vi "Deserialize Object (XML).vi"(8 "error in":errorcluster, 9 "key-value-type in":T1[](array[typedef]), 11 "object type":refnum<class "_ISerializable.lvclass">) -> (0 "casting error":errorcluster, 3 "object out":refnum<class "_ISerializable.lvclass">)   [LabVIEW 2018, in "Serializer.lvclass"]
uses:
  Serializer.lvclass
  _Serializable Base Object/_ISerializable.lvclass
  Typedefs/key-value-type cluster.ctl
  <vilib>/xml/Close Reference(Node).vi
  <resource>/objmgr/DOMUserDefRef.rc
  <vilib>/xml/NI_XML.lvlib
  <vilib>/Analysis/NI_AALBase.lvlib
  ORM Scripter/ORM Scripter.lvclass
  <vilib>/Analysis/baseanly.llb/Mean (DBL).vi
panel:
  out "error out":errorcluster
  out "XML-Pretty":string
  out "Generated XML":string
  out "default object xml string":string
  # "<Object>\n<Name>object in</Name>\n<NumLevels>2</NumLevels>\n<Class>DataTypes.lvclass</Class>\n<Version>1.0.0.4</Version>\n<Version>1.0.0.1</Version>\n<Cluster>\n</Cluster>\n<Cluster>\n<Name>DataTypes.lvclass</Name>\n<NumElts>17</NumElts>\n<Boolean>\n<Name>Boolean</Name>\n<Val>0</Val>\n</Boolean>\n<String>\n<Name>String</Name>\n<Val>STRING DATA</Val>\n</String>\n<U16>\n<Name>Ring</Name>\n<Val>1</Val>\n</U16>\n<EW>\n<Name>Enum</Name>\n<Choice>enum-value-0</Choice>\n<Choice>enum-value-1</Choice>\n<Choice>enum-value-2</Choice>\n<Val>2</Val>\n</EW>\n<DBL>\n<Name>Numeric DBL</Name>\n<Val>0.36114694623797</Val>\n</DBL>\n<SGL>\n<Name>Numeric SGL</Name>\n<Val>0.36115</Val>\n</SGL>\n<CDB>\n<Name>Numeric C-DBL</Name>\n<Val>0.36114694623797 +0.00000000000000 i</Val>\n</CDB>\n<CSG>\n<Name>Numeric C-SGL</Name>\n<Val>0.36115 +0.00000 i</Val>\n</CSG>\n<U8>\n<Name>Numeric U8</Name>\n<Val>33</Val>\n</U8>\n<I8>\n<Name>Numeric I8</Name>\n<Val>30</Val>\n</I8>\n<U16>\n<Name>Numeric U16</Name>\n<Val>28</Val>\n</U16>\n<I16>\n<Name>Numeric I16</Name>\n<Val>50</Val>\n</I16>\n<U32>\n<Name>Numeric U32</Name>\n<Val>68</Val>\n</U32>\n<I32>\n<Name>Numeric I32</Name>\n<Val>54</Val>\n</I32>\n<U64>\n<Name>Numeric U64</Name>\n<Val>45</Val>\n</U64>\n<I64>\n<Name>Numeric I64</Name>\n<Val>29</Val>\n</I64>\n<Timestamp>\n<Name>Time Stamp</Name>\n<Cluster>\n<Name></Name>\n<NumElts>4</NumElts>\n<I32>\n<Name></Name>\n<Val>0</Val>\n</I32>\n<I32>\n<Name></Name>\n<Val>632510464</Val>\n</I32>\n<I32>\n<Name></Name>\n<Val>-640183486</Val>\n</I32>\n<I32>\n<Name></Name>\n<Val>0</Val>\n</I32>\n</Cluster>\n</Timestamp>\n</Cluster>\n</Object>"
  # "<Object>\n<Name>object type</Name>\n<NumLevels>2</NumLevels>\n<Class>DataTypes.lvclass</Class>\n<Version>1.0.0.4</Version>\n<Version>1.0.0.1</Version>\n<Cluster>\n<Name>DataTypes.lvclass</Name>\n<NumElts>17</NumElts>\n<Boolean>\n<Name>Boolean</Name>\n<Val>0</Val>\n</Boolean>\n<String>\n<Name>String</Name>\n<Val>STRING DATA</Val>\n</String>\n<U16>\n<Name>Ring</Name>\n<Val>1</Val>\n</U16>\n<EW>\n<Name>Enum</Name>\n<Choice>enum-value-0</Choice>\n<Choice>enum-value-1</Choice>\n<Choice>enum-value-2</Choice>\n<Val>2</Val>\n</EW>\n<DBL>\n<Name>Numeric DBL</Name>\n<Val>0.69305757967832</Val>\n</DBL>\n<SGL>\n<Name>Numeric SGL</Name>\n<Val>0.69306</Val>\n</SGL>\n<CDB>\n<Name>Numeric C-DBL</Name>\n<Val>0.69305757967832 +0.00000000000000 i</Val>\n</CDB>\n<CSG>\n<Name>Numeric C-SGL</Name>\n<Val>0.69306 +0.00000 i</Val>\n</CSG>\n<U8>\n<Name>Numeric U8</Name>\n<Val>90</Val>\n</U8>\n<I8>\n<Name>Numeric I8</Name>\n<Val>84</Val>\n</I8>\n<U16>\n<Name>Numeric U16</Name>\n<Val>4</Val>\n</U16>\n<I16>\n<Name>Numeric I16</Name>\n<Val>41</Val>\n</I16>\n<U32>\n<Name>Numeric U32</Name>\n<Val>91</Val>\n</U32>\n<I32>\n<Name>Numeric I32</Name>\n<Val>70</Val>\n</I32>\n<U64>\n<Name>Numeric U64</Name>\n<Val>48</Val>\n</U64>\n<I64>\n<Name>Numeric I64</Name>\n<Val>30</Val>\n</I64>\n<Timestamp>\n<Name>Time Stamp</Name>\n<Val>\n</Val>\n</Timestamp>\n</Cluster>\n</Object>"
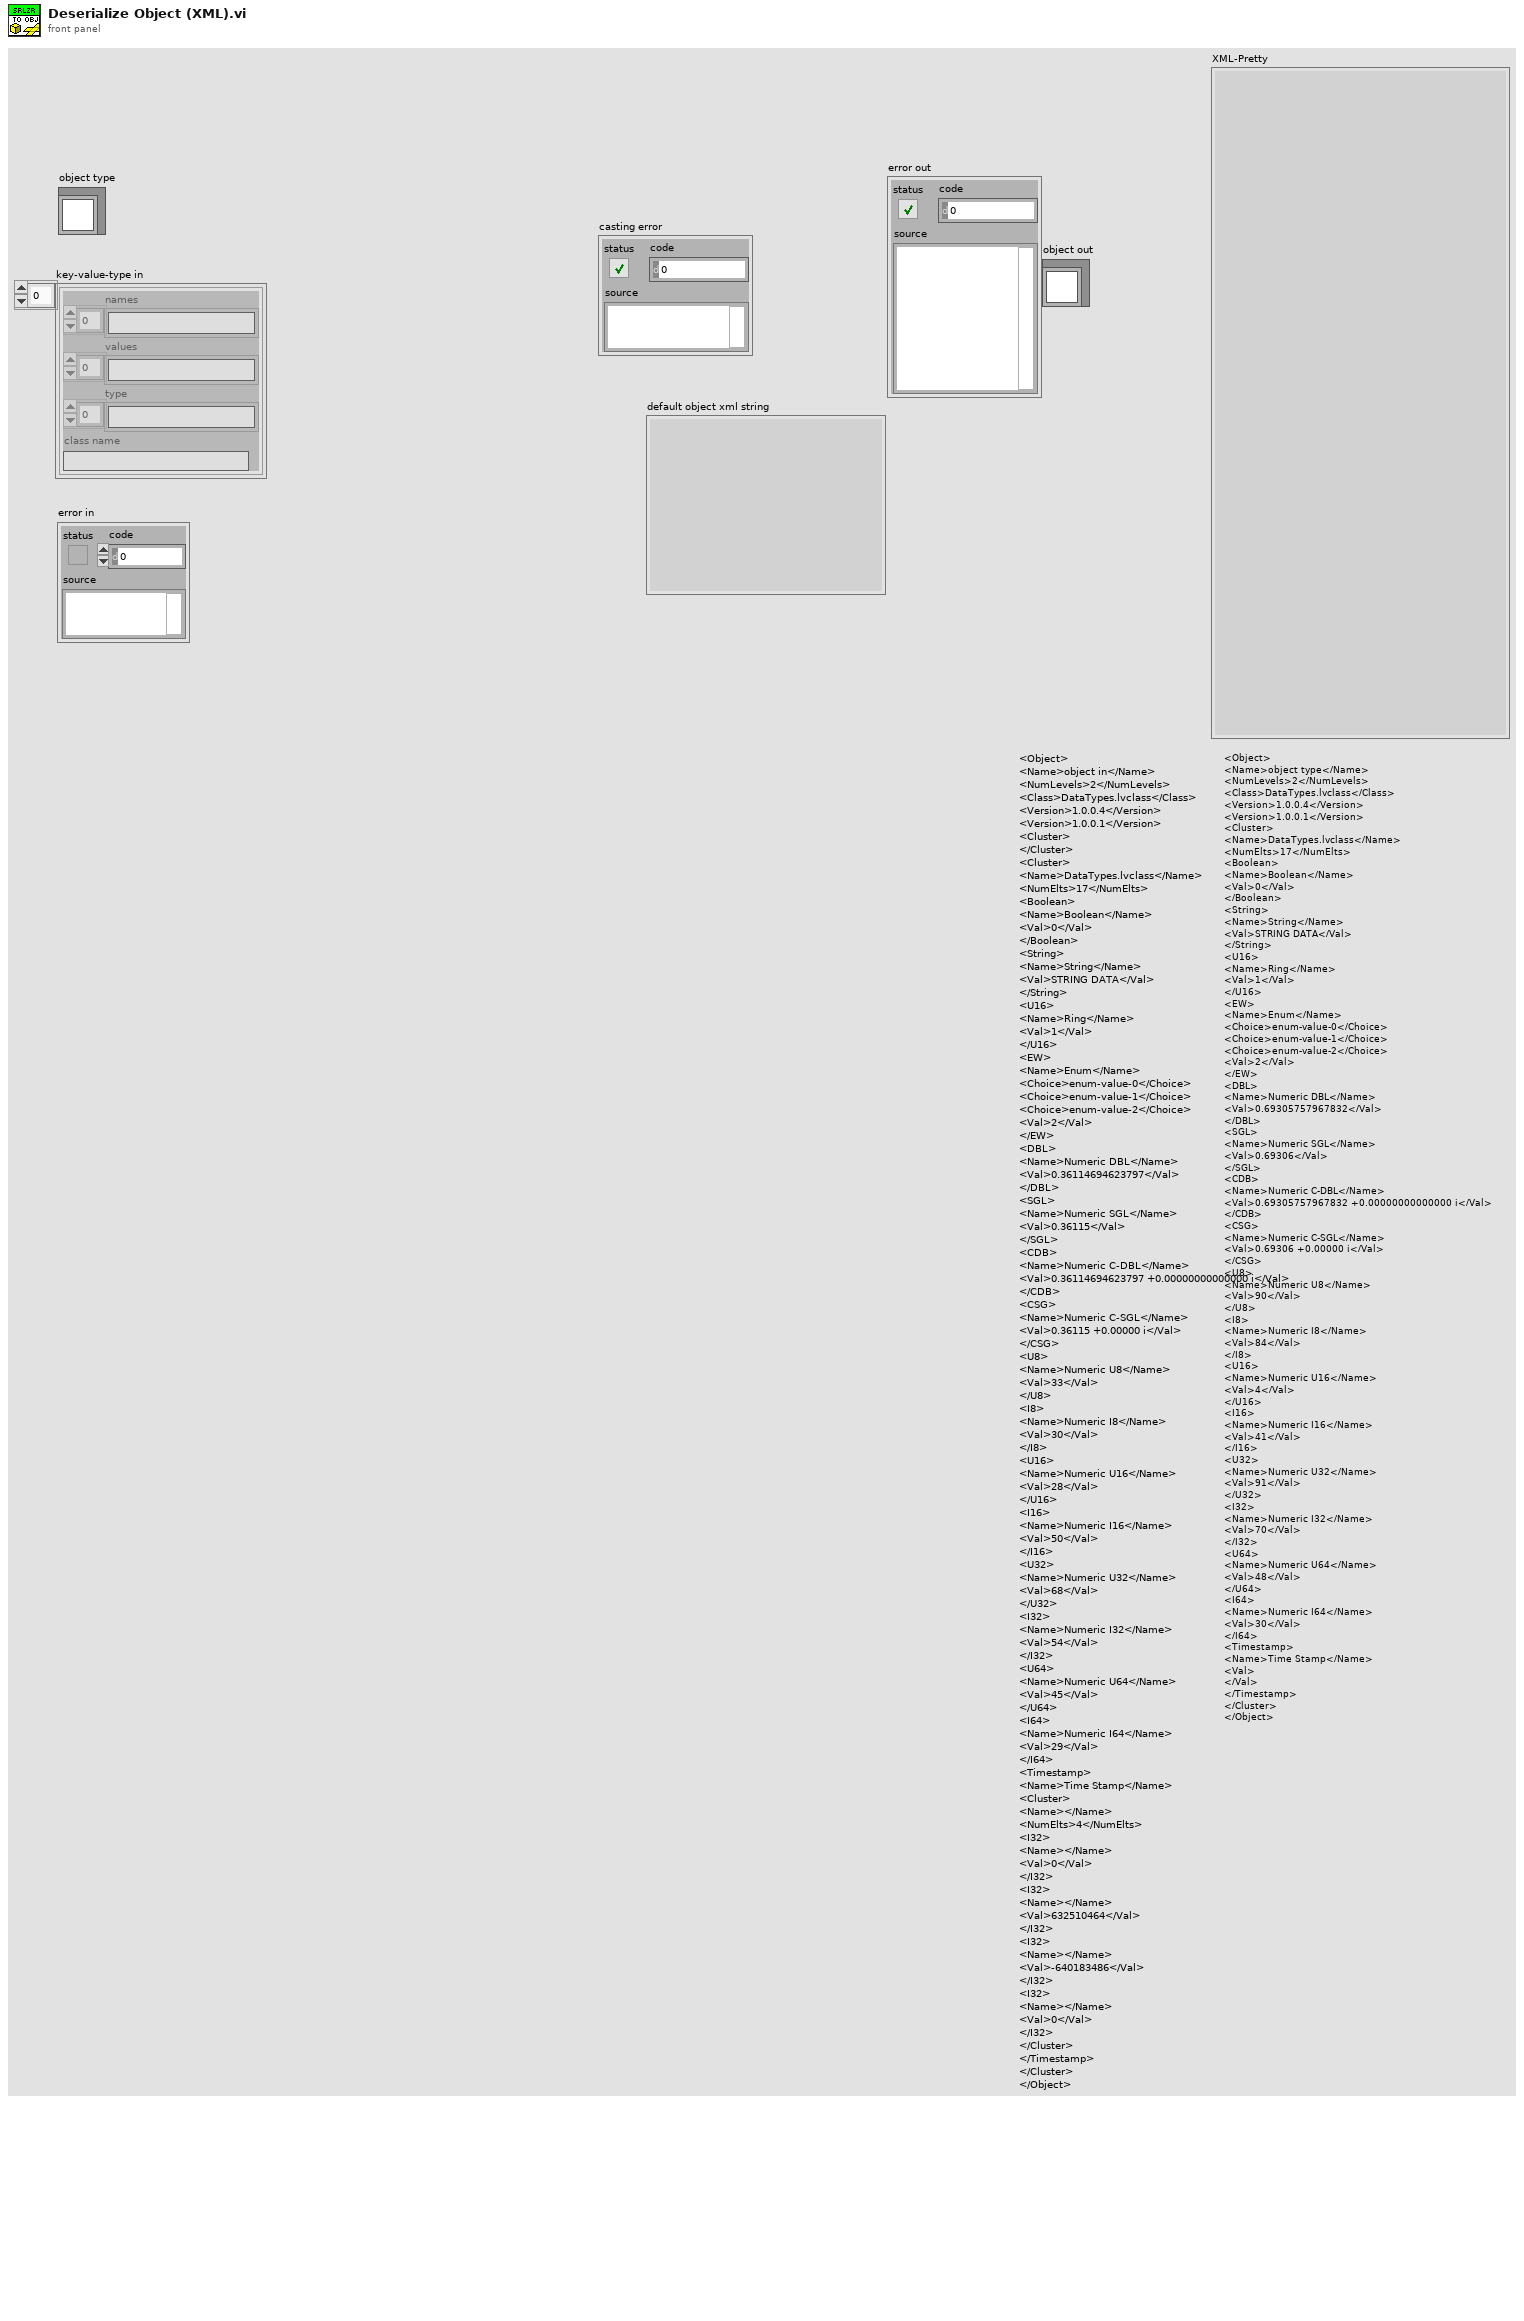
[diagram p1: front panel]
types:
  T1 = typedef "key-value-type cluster.ctl" = cluster{"names":string[], "values":string[], "type":string[], "class name":string}
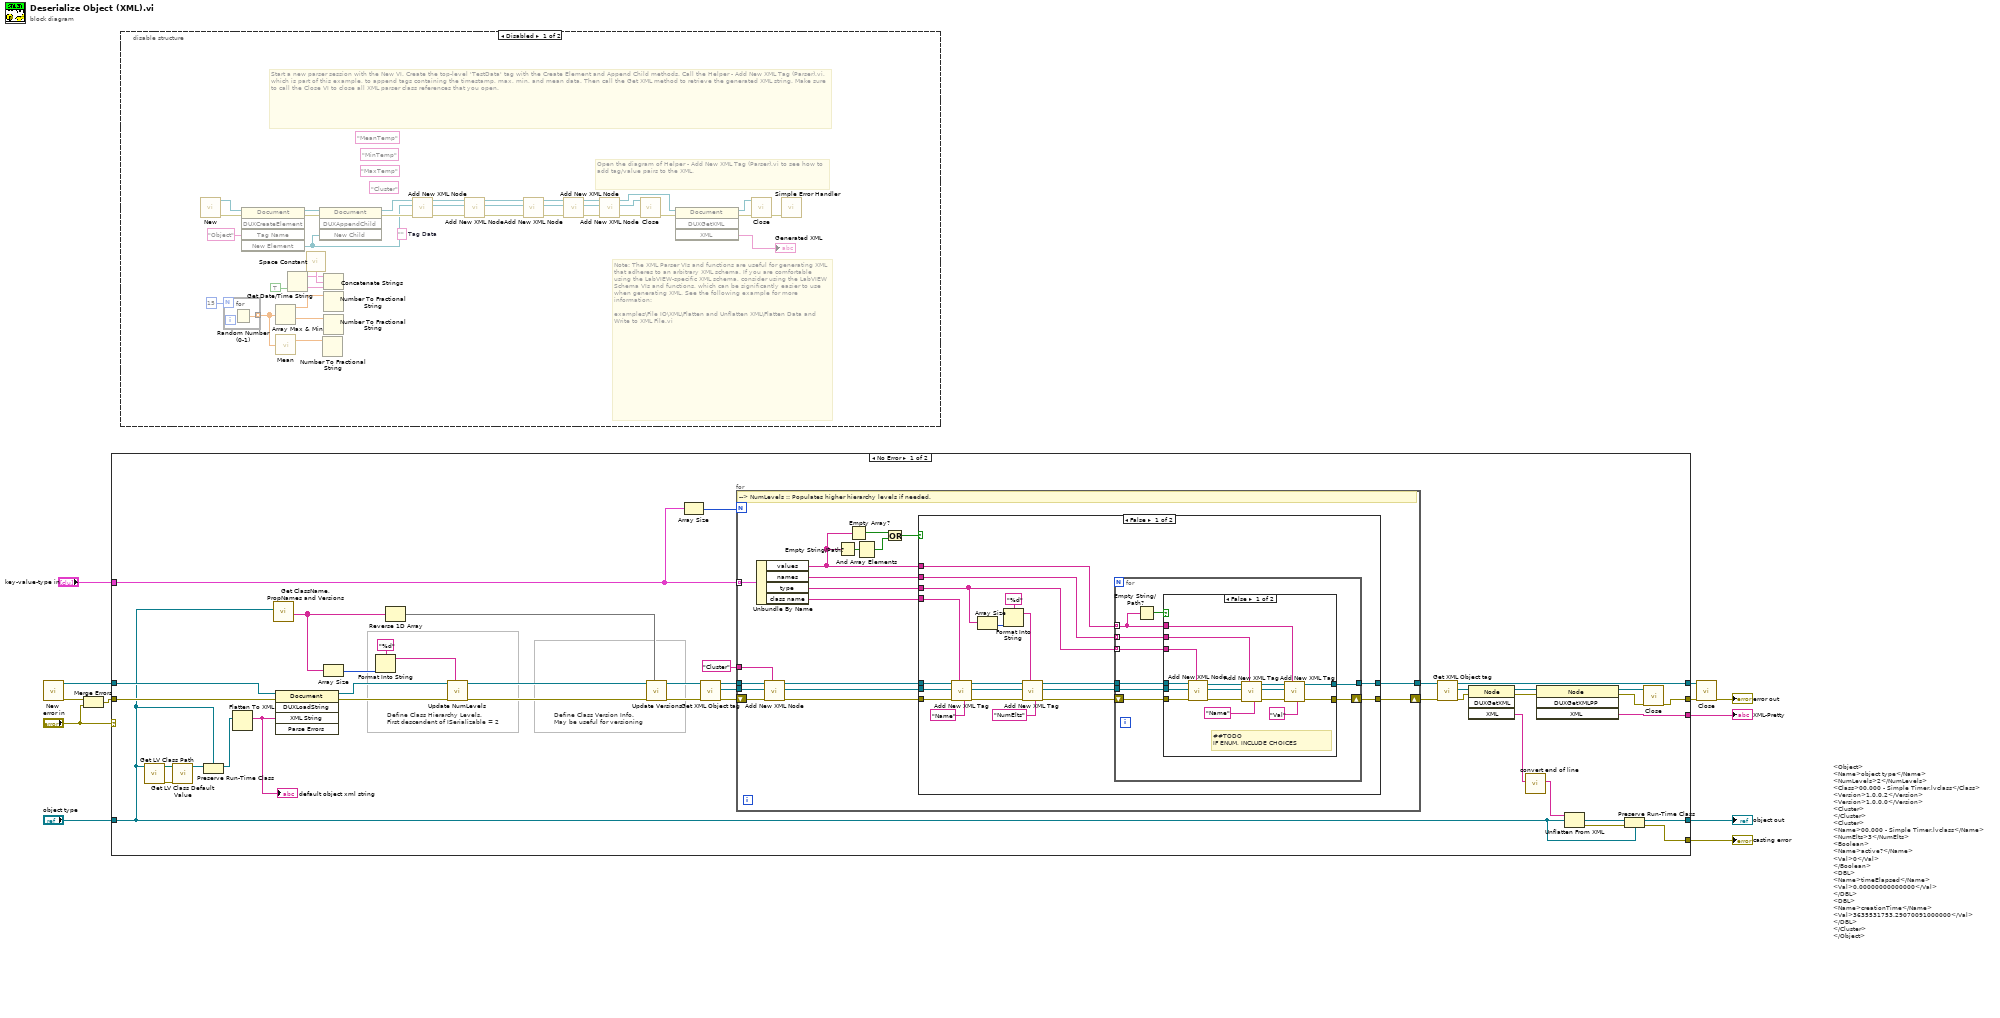
[diagram p0: block diagram]
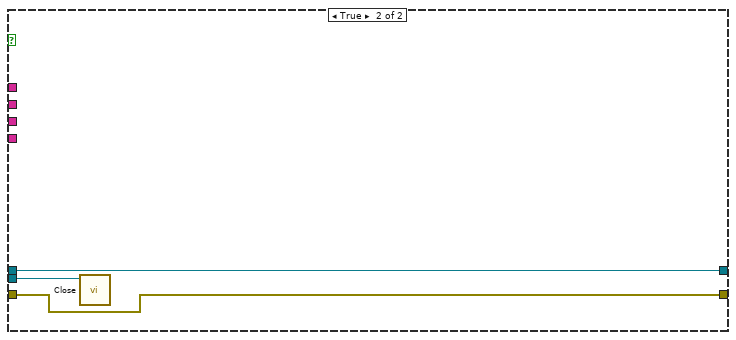
[diagram p3: hidden frame]
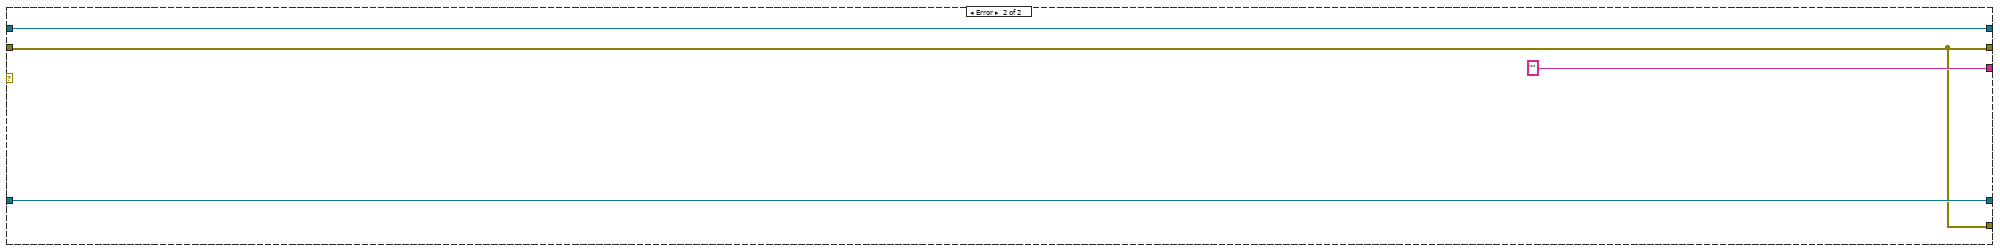
[diagram p4: hidden frame]
diagram:
  # "<Object>\n<Name>object type</Name>\n<NumLevels>2</NumLevels>\n<Class>00.000 - Simple Timer.lvclass</Class>\n<Version>1.0.0.2</Version>\n<Version>1.0.0.0</Version>\n<Cluster>\n</Cluster>\n<Cluster>\n<Name>00.000 - Simple Timer.lvclass</Name>\n<NumElts>3</NumElts>\n<Boolean>\n<Name>active?</Name>\n<Val>0</Val>\n</Boolean>\n<DBL>\n<Name>timeElapsed</Name>\n<Val>0.00000000000000</Val>\n</DBL>\n<DBL>\n<Name>creationTime</Name>\n<Val>3635531753.29070091000000</Val>\n</DBL>\n</Cluster>\n</Object>"
  n1 = call <vilib>:"New.vi"() -> ("error out"=w7:errorcluster, "DOM document out"=w11:refnum<k20>)  [unwired: 8 in]
  n2 = Merge Errors(w7, "error in") -> (w6:errorcluster)
  n3 = case shown="No Error" "error in" {
    tunnel: [w26 w126] -> w2
    tunnel: "object type" -> [w23 w126]
    tunnel: w11 -> [w53 w125]
    tunnel: w6 -> [w54 w123]
    tunnel: [w24 w125] -> w10
    tunnel: [w29 w123] -> w9
    tunnel: [w25 ""] -> w4
    tunnel: "key-value-type in" -> [w17 _]
    tunnel: [w16 w123] -> w1
    frame No Error {
      # "Define Class Version Info.\nMay be useful for versioning"
      # "Define Class Hierarchy Levels.\nFirst descendent of ISerializable = 2"
      n4 = call <vilib>:"Get LV Class Path.vi"("object"=w23) -> ("error out"=w51:errorcluster, "class path"=w52:path)  [unwired: 9 in]
      n5 = call <vilib>:"Get LV Class Default Value.vi"("error in (no error)"=w51, "class path"=w52) -> ("object"=w48:refnum<class>)  [unwired: 8 in, 1 out]
      n6 = Preserve Run-Time Class(object in=w48, 2:w23) -> (object out=w47:refnum<class "_ISerializable.lvclass">)  [unwired: 1 in, 1 out]
      n7 = Flatten To XML(anything=w47) -> (xml string=w49:string)
      "default object xml string" <- w49
      n8 = call "Get ClassName, PropNames and Versions.vi"("object"=w23) -> ("versions"=w19:string[])  [unwired: 9 in, 1 out]
      n9 = invoke class="Document" method="DUXLoadString"(reference=w53, error in=w54, "XML String"=w49) -> (reference out=w46:refnum<k20>, error out=w50:errorcluster)  [unwired: 2 in, 3 out]
      n10 = Array Size(array=w19) -> (size(s)=w22:i32)
      n11 = Format Into String(format string="%d", w22) -> (resulting string=w20:string)  [unwired: 2 in, 1 out]
      n12 = Reverse 1D Array(array=w19) -> (reversed array=w18:string[])
      n13 = call "Update NumLevels.vi"("NumLevels"=w20, "error in"=w50, "Refnum in"=w46) -> ("error out"=w44:errorcluster, "Refnum out"=w45:refnum<k20>)  [unwired: 7 in]
      n14 = call "Update Versions.vi"("Versions"=w18, "error in"=w44, "Refnum in"=w45) -> ("error out"=w42:errorcluster, "Refnum out"=w43:refnum<k20>)  [unwired: 7 in]
      n15 = Array Size(array=w17) -> (size(s)=w28:i32)
      n16 = call "Get XML Object tag.vi"("error in (no error)"=w42, "Refnum in"=w43) -> ("error out"=w39:errorcluster, "FirstChild"=w40:refnum<k20>, "Refnum out"=w41:refnum<k20>)  [unwired: 7 in]
      n17 = for {
        N: w28 -> [_]
        tunnel: w40 -> [w70]
        tunnel: w41 -> [w71]
        tunnel: [w72] -> w36
        shift-right: [w67] -> w35
        shift-left: w39 -> [w69]
        tunnel: "Cluster" ("Qualified Name") -> [w68]
        tunnel: w17 -> [w66] mode=indexing
        # "--> NumLevels :: Populates higher hierarchy levels if needed."
        n18 = Unbundle By Name(w66) -> ("values"=w55:string[], "names"=w65:string[], "type"=w64:string[], "class name"=w62:string)
        n19 = call "Add New XML Node.vi"("Node Name"=w68, "error in"=w69, "Owning Element"=w70, "DOM doc"=w71) -> ("error out"=w63:errorcluster, "new element"=w60:refnum<k20>, "DOM doc out"=w61:refnum<k20>)  [unwired: 5 in]
        n20 = Empty String/Path?(string/path=w55) -> (empty?=w59:bool[])
        n21 = Empty Array?(array=w55) -> (empty?=w58:bool)
        n22 = And Array Elements(Boolean array=w59) -> (logical AND=w57:bool)
        n23 = Or(x=w58, y=w57) -> (x .or. y?=w56:bool)
        n24 = case shown="False" w56 {
          tunnel: [w90 w122] -> w72
          tunnel: [w89 w121] -> w67
          tunnel: w65 -> [w88 _]
          tunnel: w55 -> [w87 _]
          tunnel: w64 -> [w86 _]
          tunnel: w63 -> [w83 w121]
          tunnel: w62 -> [w82 _]
          tunnel: w61 -> [w80 w122]
          tunnel: w60 -> [w75 w120]
          frame False {
            n25 = call "Add New XML Tag.vi"("Tag Name"="Name" ("Qualified Name"), "Tag Data"=w82, "error in (no error)"=w83, "Owning Element"=w75, "DOM document"=w80) -> ("error out"=w81:errorcluster, "dup Owning Element"=w76:refnum<k20>, "dup DOM document"=w77:refnum<k20>)  [unwired: 4 in]
            n26 = Array Size(array=w86) -> (size(s)=w91:i32)
            n27 = Format Into String(format string="%d", w91) -> (resulting string=w85:string)  [unwired: 2 in, 1 out]
            n28 = call "Add New XML Tag.vi"("Tag Name"="NumElts", "Tag Data"=w85, "error in (no error)"=w81, "Owning Element"=w76, "DOM document"=w77) -> ("error out"=w84:errorcluster, "dup Owning Element"=w78:refnum<k20>, "dup DOM document"=w79:refnum<k20>)  [unwired: 4 in]
            n29 = for {
              tunnel: w79 -> [w101]
              shift-right: [w96] -> w89
              shift-left: w84 -> [w99]
              tunnel: w86 -> [w98] mode=indexing
              tunnel: [w95] -> w90
              tunnel: w88 -> [w97] mode=indexing
              tunnel: w87 -> [w93] mode=indexing
              tunnel: w78 -> [w100]
              n30 = Empty String/Path?(string/path=w93) -> (empty?=w94:bool)
              n31 = case shown="False" w94 {
                tunnel: w101 -> [w117 w119]
                tunnel: w100 -> [w116 _]
                tunnel: w99 -> [w115 w118]
                tunnel: w98 -> [w114 _]
                tunnel: w97 -> [w113 _]
                tunnel: [w110 w118] -> w96
                tunnel: [w109 w119] -> w95
                tunnel: w93 -> [w107 _]
                frame False {
                  # "##TODO\nIF ENUM, INCLUDE CHOICES"
                  n32 = call "Add New XML Node.vi"("Node Name"=w114, "error in"=w115, "Owning Element"=w116, "DOM doc"=w117) -> ("error out"=w112:errorcluster, "new element"=w108:refnum<k20>, "DOM doc out"=w104:refnum<k20>)  [unwired: 5 in]
                  n33 = call "Add New XML Tag.vi"("Tag Name"="Name", "Tag Data"=w113, "error in (no error)"=w112, "Owning Element"=w108, "DOM document"=w104) -> ("error out"=w111:errorcluster, "dup Owning Element"=w106:refnum<k20>, "dup DOM document"=w105:refnum<k20>)  [unwired: 4 in]
                  n34 = call "Add New XML Tag.vi"("Tag Name"="Val", "Tag Data"=w107, "error in (no error)"=w111, "Owning Element"=w106, "DOM document"=w105) -> ("error out"=w110:errorcluster, "dup DOM document"=w109:refnum<k20>)  [unwired: 4 in, 1 out]
                }
                frame True {
                }
              }
            }
          }
          frame True {
            n35 = call-poly <vilib>:"Close.vi"("node"=w120) -> ()  [unwired: 1 in, 8 out]
          }
        }
      }
      n36 = call "Get XML Object tag.vi"("error in (no error)"=w35, "Refnum in"=w36) -> ("error out"=w33:errorcluster, "FirstChild"=w34:refnum<k20>, "Refnum out"=w24:refnum<k20>)  [unwired: 7 in]
      n37 = invoke class="Node" method="DUXGetXML"(reference=w34, error in=w33) -> (reference out=w32:refnum<k20>, error out=w31:errorcluster, "XML"=w13:string)  [unwired: 2 in, 1 out]
      n38 = call "convert end of line.vi"("XML"=w13) -> ("String"=w14:string)  [unwired: 10 in]
      n39 = invoke class="Node" method="DUXGetXMLPP"(reference=w32, error in=w31) -> (reference out=w37:refnum<k20>, error out=w30:errorcluster, "XML"=w25:string)  [unwired: 2 in, 1 out]
      n40 = Unflatten From XML(xml string=w14, type=w23) -> (value=w27:refnum<class "_ISerializable.lvclass">, error out=w15:errorcluster)  [unwired: 1 in]
      n41 = Preserve Run-Time Class(object in=w27, error in=w15, 2:w23) -> (object out=w26:refnum<class "_ISerializable.lvclass">, error out=w16:errorcluster)
      n42 = call-poly <vilib>:"Close.vi"("error in (no error)"=w30, "node"=w37) -> ("error out"=w29:errorcluster)  [unwired: 7 in]
    }
    frame Error {
    }
  }
  "object out" <- w2
  "XML-Pretty" <- w4
  "casting error" <- w1
  n43 = disable-structure shown="Disabled" {
    frame Disabled {
      (unwired) ""  # Tag Data
      (unwired) "MeanTemp" ("Tag Name")
      (unwired) "MinTemp" ("Tag Name")
      (unwired) "MaxTemp" ("Tag Name")
      (unwired) "Cluster" ("Tag Name")
      # "Note: The XML Parser VIs and functions are useful for generating XML that adheres to an arbitrary XML schema. If you are comfortable using the LabVIEW-specific XML schema, consider using the LabVIEW Schema VIs and functions, which can be significantly easier to use when generating XML. See the following example for more information:\n\nexamples\\File IO\\XML\\Flatten and Unflatten XML\\Flatten Data and Write to XML File.vi"
      # "Open the diagram of Helper - Add New XML Tag (Parser).vi to see how to add tag/value pairs to the XML."
      # "Start a new parser session with the New VI. Create the top-level 'TestData' tag with the Create Element and Append Child methods. Call the Helper - Add New XML Tag (Parser).vi, which is part of this example, to append tags containing the timestamp, max, min, and mean data. Then call the Get XML method to retrieve the generated XML string. Make sure to call the Close VI to close all XML parser class references that you open."
      n44 = call <vilib>:"New.vi"() -> ("error out"=w149:errorcluster, "DOM document out"=w146:refnum<k20>)  [unwired: 1 in, 7 out]
      n45 = for {
        N: 15 -> [_]
        tunnel: [w163] -> w154 mode=indexing
        n46 = Random Number (0-1)() -> (number: 0 to 1=w163:dbl)
      }
      n47 = invoke class="Document" method="DUXCreateElement"(reference=w146, error in=w149, "Tag Name"="Object" ("Qualified Name")) -> (reference out=w150:refnum<k20>, error out=w148:errorcluster, "New Element"=w133:refnum<k20>)  [unwired: 2 in, 2 out]
      n48 = Array Max & Min ("Max & Min")(array=w154) -> (max value=w131:dbl, min value=w132:dbl)  [unwired: 2 out]
      n49 = call-poly <vilib>:"Mean.vi"("X"=w154) -> ("mean"=w152:dbl)  [unwired: 1 out]
      n50 = Get Date/Time String(want seconds? (F)=TRUE) -> (date string=w160:string, time string=w159:string)  [unwired: 2 out]
      n51 = call <vilib>:"Space Constant.vi"() -> ("String"=w161:string)
      n52 = invoke class="Document" method="DUXAppendChild"(reference=w150, error in=w148, "New Child"=w133) -> (reference out=w136:refnum<k20>, error out=w135:errorcluster)  [unwired: 1 in, 2 out]
      n53 = Number To Fractional String(number=w152) -> ()  [unwired: 4 out]
      n54 = Concatenate Strings(w160, w161, w159) -> ()  [unwired: 1 out]
      n55 = Number To Fractional String(number=w131) -> ()  [unwired: 4 out]
      n56 = Number To Fractional String(number=w132) -> ()  [unwired: 4 out]
      n57 = call "Add New XML Node.vi"("error in"=w135, "Owning Element"=w133, "DOM doc"=w136) -> ("error out"=w134:errorcluster, "new element"=w129:refnum<k20>, "DOM doc out"=w130:refnum<k20>)  [unwired: 6 in]
      n58 = call "Add New XML Node.vi"("Owning Element"=w129, "DOM doc"=w130) -> ("new element"=w127:refnum<k20>, "DOM doc out"=w128:refnum<k20>)  [unwired: 7 in, 1 out]
      n59 = call "Add New XML Node.vi"("error in"=w134, "Owning Element"=w127, "DOM doc"=w128) -> ("error out"=w139:errorcluster, "new element"=w137:refnum<k20>, "DOM doc out"=w138:refnum<k20>)  [unwired: 6 in]
      n60 = call "Add New XML Node.vi"("error in"=w139, "Owning Element"=w137, "DOM doc"=w138) -> ("error out"=w142:errorcluster, "new element"=w141:refnum<k20>, "DOM doc out"=w140:refnum<k20>)  [unwired: 6 in]
      n61 = call "Add New XML Node.vi"("error in"=w142, "Owning Element"=w141, "DOM doc"=w140) -> ("error out"=w145:errorcluster, "new element"=w143:refnum<k20>, "DOM doc out"=w144:refnum<k20>)  [unwired: 6 in]
      n62 = call-poly <vilib>:"Close.vi"("error in (no error)"=w145, "node"=w143) -> ("error out"=w155:errorcluster)  [unwired: 7 out]
      n63 = invoke class="Document" method="DUXGetXML"(reference=w144, error in=w155) -> (reference out=w156:refnum<k20>, error out=w158:errorcluster, "XML"=→"Generated XML":string)  [unwired: 2 in, 1 out]
      n64 = call-poly <vilib>:"Close.vi"("error in (no error)"=w158, "node"=w156) -> ("error out"=w147:errorcluster)  [unwired: 7 out]
      n65 = call <vilib>:"Simple Error Handler.vi"("error in (no error)"=w147) -> ()  [unwired: 1 in, 8 out]
    }
    frame Enabled {
    }
  }
  n66 = call-poly <vilib>:"Close.vi"("error in (no error)"=w9, "node"=w10) -> ("error out"=→"error out":errorcluster)  [unwired: 7 in]
